vi "check_boc_rms_amplitude_char.vi"(8 "error in (no error)":errorcluster, 9 "Amplitude (1.0 Vpp)":dbl[](array[numeric]) format="%#.4f", 10 "Frequency (Hz)":dbl=1.0 format="%#.4f", 11 "app_data in":T2) -> (0 "error out":errorcluster, 1 "meas":dbl[][](array[numeric]), 2 "boc_data":sgl[][](array[numeric]), 3 "app_data_out":T2)   [LabVIEW 2017]
uses:
  controls/app_data.ctl
  controls/instruments.ctl
  Unicorn Labview Library/Control/unicorn_Param.ctl
  Unicorn Labview Library/Control/unicorn_conn.ctl
  Unicorn Labview Library/Control/unicorn_JSON.ctl
  Unicorn Labview Library/Control/unicorn_ParamInt.ctl
  Unicorn Labview Library/Control/unicorn_Telemetry.ctl
  Unicorn Labview Library/Control/unicorn_Table.ctl
  Unicorn Labview Library/Control/unicorn_ParamFloat.ctl
  controls/attenuator_dB.ctl
  Unicorn Labview Library/Unicorn Library.lvlib
panel:
  out "Attenuator(dB)":T1
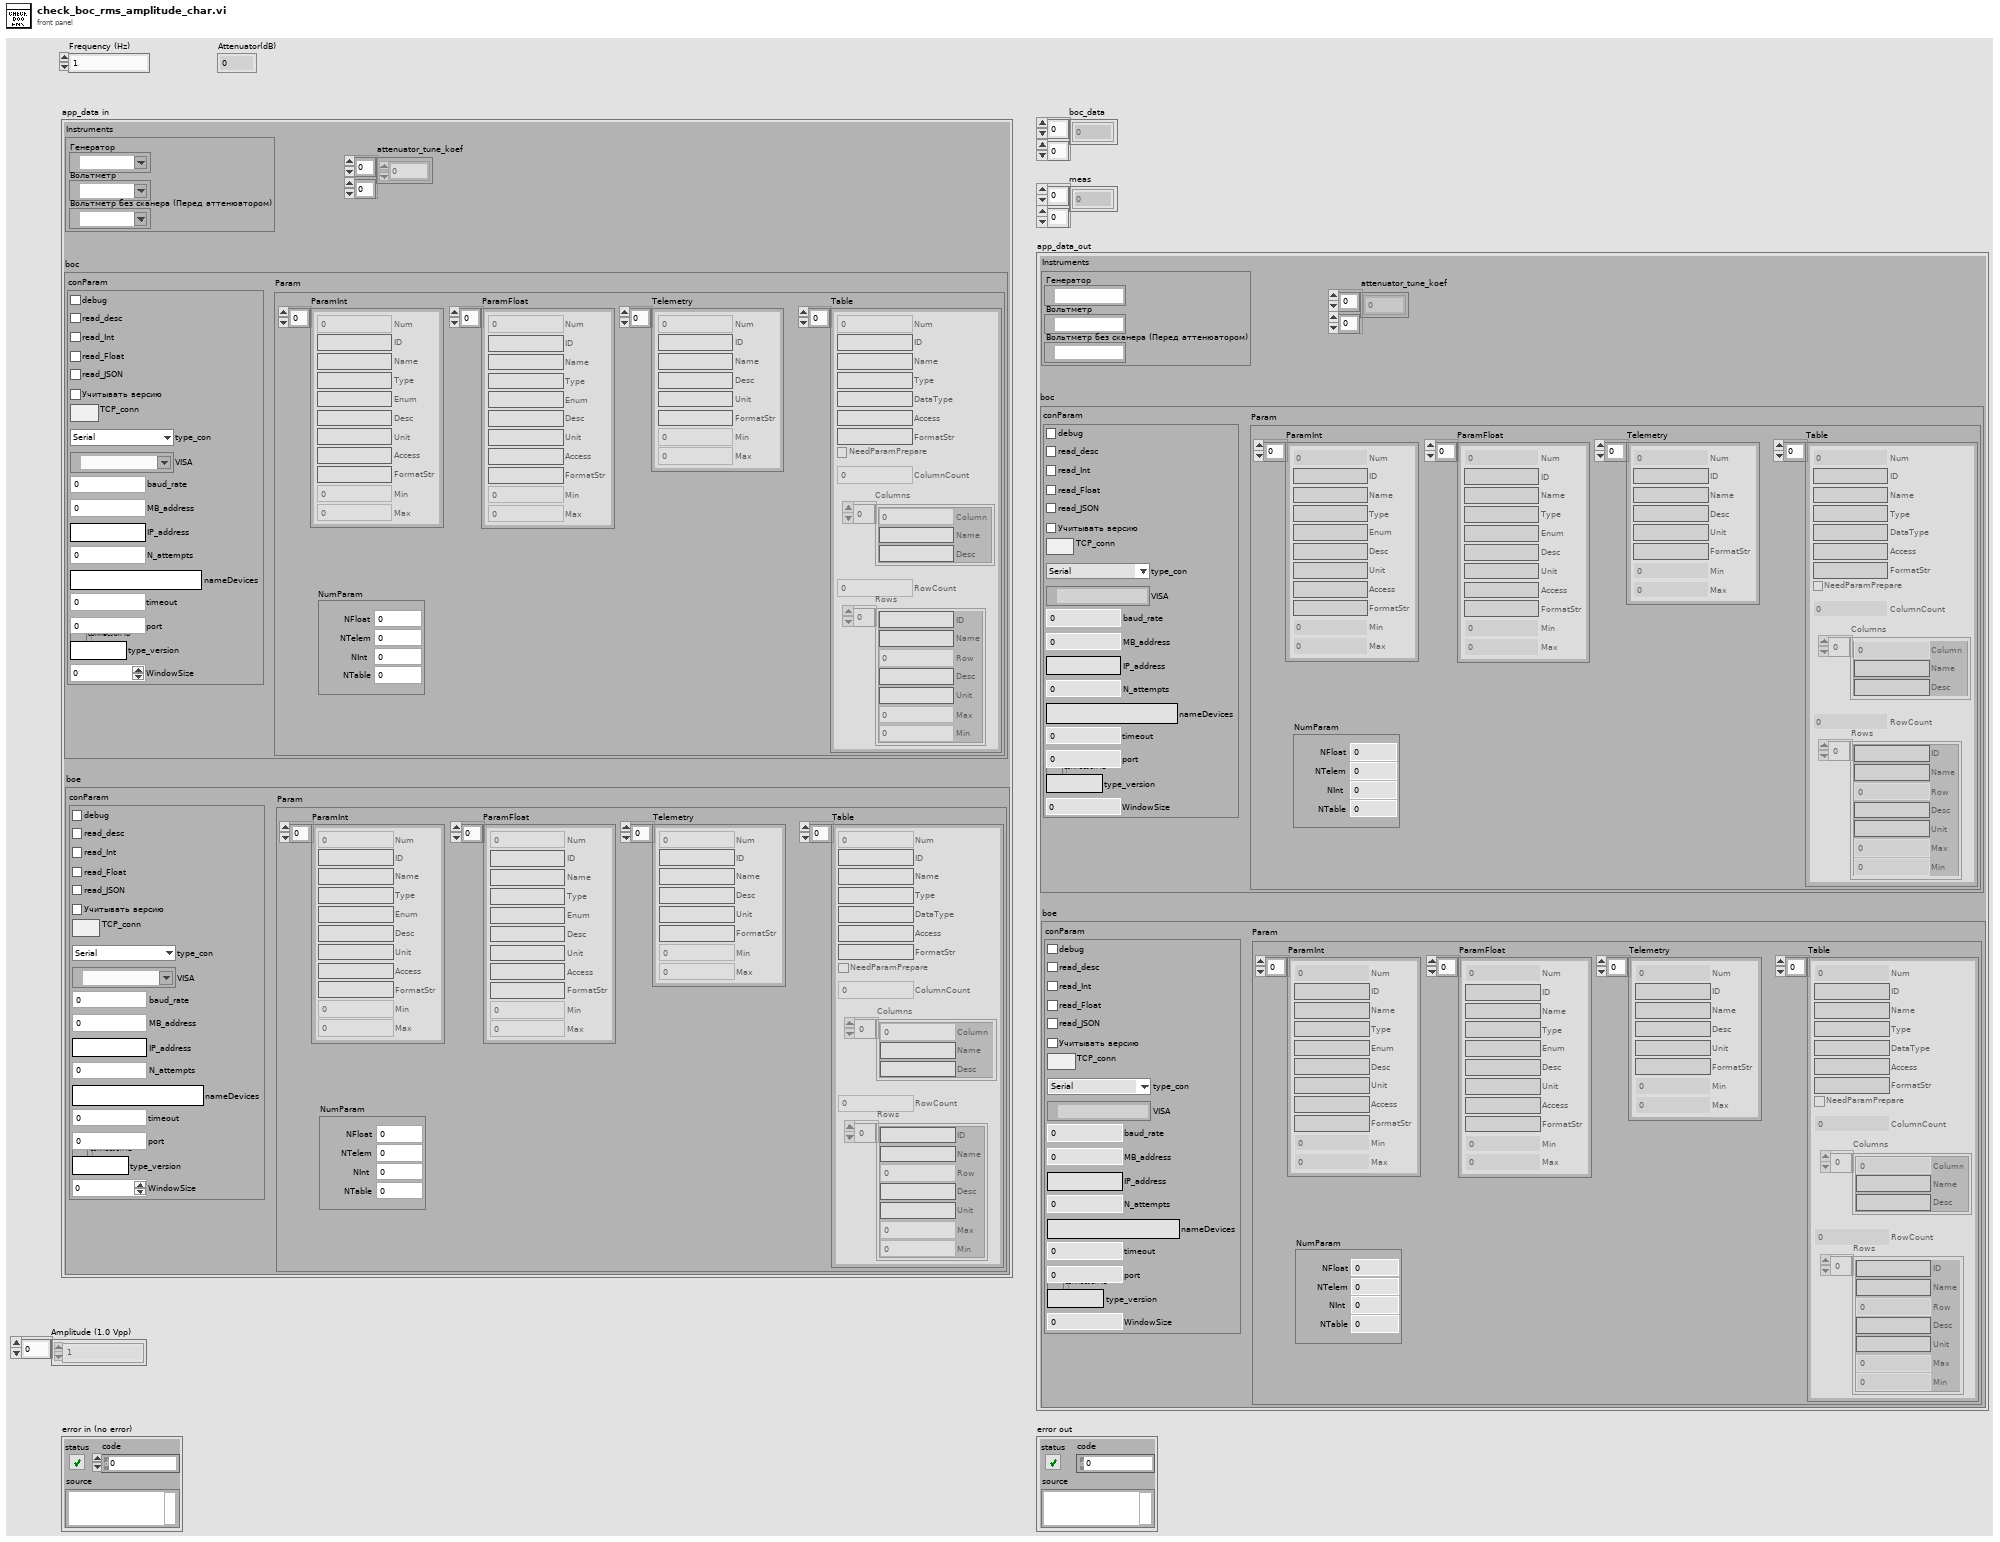
[diagram p1: front panel]
types:
  T1 = typedef "attenuator_dB.ctl" = enum16{"0", "20", "40", "60"}
  T2 = typedef "app_data.ctl" = cluster{"Instruments":T3, "boc":T4, "boe":T4, "attenuator_tune_koef":dbl[][]}
  T3 = typedef "instruments.ctl" = cluster{"generator":refnum<visa-resource-name>, "voltment_with_scaner":refnum<visa-resource-name>, "voltment_without_scaner":refnum<visa-resource-name>}
  T4 = typedef "Unicorn Library.lvlib/unicorn_Param.ctl" = cluster{"conParam":T5, "Param":T6}
  T5 = typedef "Unicorn Library.lvlib/unicorn_conn.ctl" = cluster{"ReadIntParam":bool, "ReadDescrParam":bool, "ReadFloatParam":bool, "debug":bool, "ReadJSON":bool, "IP_address":string, "N_attempts":i32, "type_con":enum16{"Serial", "TCP"}, "MB_address":i32, "VISA":refnum<visa-resource-name>, "connection ID":refnum<k5>, "nameDevices":string, "timeout":i32, "port":u16, "type_version":string, "baud_rate":u32, "VersionControl":bool, "TCP_conn":bool, "WindowSize":i32}
  T6 = typedef "Unicorn Library.lvlib/unicorn_JSON.ctl" = cluster{"NumParam":cluster{"NTelem":i32, "NInt":i32, "NFloat":i32, "NTable":i32}, "ParamInt":T7, "Telemetry":T8, "Table":T9, "ParamFloat":T10}
  T7 = typedef "Unicorn Library.lvlib/unicorn_ParamInt.ctl" = cluster{"ID":string, "Num":i32, "Name":string, "Type":string, "Enum":string, "Desc":string, "Unit":string, "Access":string, "FormatStr":string, "Min":i32, "Max":i32}[]
  T8 = typedef "Unicorn Library.lvlib/unicorn_Telemetry.ctl" = cluster{"ID":string, "Num":i32, "Name":string, "Desc":string, "Unit":string, "FormatStr":string, "Min":i32, "Max":i32}[]
  T9 = typedef "Unicorn Library.lvlib/unicorn_Table.ctl" = cluster{"Num":i32, "Access":string, "ColumnCount":i32, "NeedParamPrepare":bool, "Columns":cluster{"Column":i32, "Desc":string, "Name":string}[], "DataType":string, "FormatStr":string, "ID":string, "Name":string, "RowCount":i32, "Rows":cluster{"Desc":string, "ID":string, "Max":i32, "Min":i32, "Name":string, "Row":i32, "Unit":string}[], "Type":string}[]
  T10 = typedef "Unicorn Library.lvlib/unicorn_ParamFloat.ctl" = cluster{"ID":string, "Num":i32, "Name":string, "Type":string, "Enum":string, "Desc":string, "Unit":string, "Access":string, "FormatStr":string, "Min":i32, "Max":i32}[]
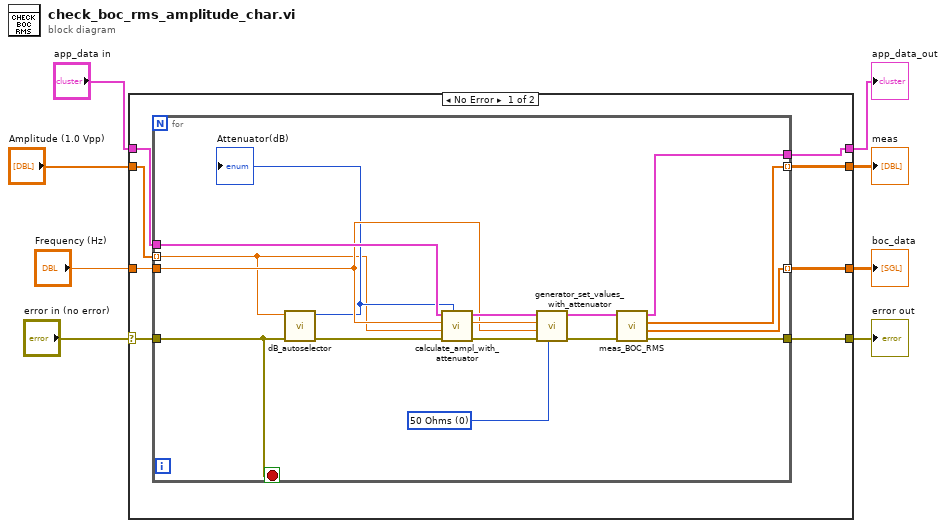
[diagram p0: block diagram]
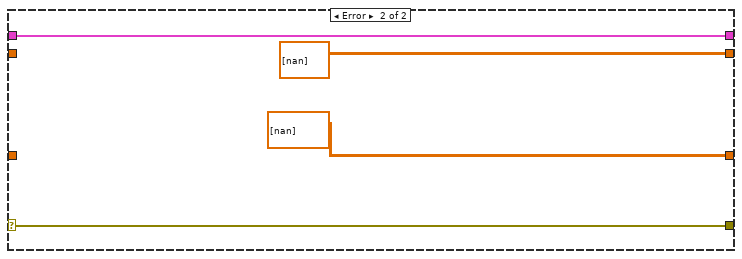
[diagram p2: hidden frame]
diagram:
  n1 = case shown="No Error" "error in (no error)" {
    selector: "error in (no error)" -> [w9 w36]
    tunnel: [w16 dbl[][] [[nan]] ("meas")] -> w8
    tunnel: [w15 sgl[][] [[nan]] ("boc_data")] -> w7
    tunnel: [w14 w36] -> w6
    tunnel: [w13 w35] -> w5
    tunnel: "Amplitude (1.0 Vpp)" -> [w12 _]
    tunnel: "app_data in" -> [w11 w35]
    tunnel: "Frequency (Hz)" -> [w10 _]
    frame No Error {
      n2 = for {
        tunnel: [w28] -> w16 mode=indexing
        tunnel: [w27] -> w15 mode=indexing
        tunnel: w9 -> [w17]
        tunnel: [w29] -> w14
        tunnel: w11 -> [w26]
        tunnel: [w30] -> w13
        tunnel: w12 -> [w19] mode=indexing
        tunnel: w10 -> [w21]
        stop <- w17 stop-if-true
        w22 = u16 0 items=["50 Ohms", "High Impedance"] ("Impedance (0: 50 Ohms)")
        n3 = call "dB_autoselector.vi"("error_in"=w17, "Amplitude"=w19) -> ("error_out"=w18:errorcluster, "Attenuator(dB)"=w20:T1)  [unwired: 8 in]
        "Attenuator(dB)" <- w20
        n4 = call "calculate_ampl_with_attenuator.vi"("Attenuator(dB)"=w20, "error in"=w18, "Amplitude_in"=w19, "frequency"=w21, "app_data in in"=w26) -> ("error out"=w25:errorcluster, "Amplitude_out"=w24:dbl, "app_data out"=w23:T2)  [unwired: 4 in]
        n5 = call "generator_set_values_with_attenuator.vi"("Impedance (0: 50 Ohms)"=w22, "error in (no error)"=w25, "Frequency (1000 Hz)"=w21, "Amplitude (1.0 Vpp)"=w24, "app_data"=w23) -> ("error out"=w31:errorcluster, "output cluster"=w32:T2)  [unwired: 5 in]
        n6 = call "meas_BOC_RMS.vi"("error in (no error)"=w31, "output cluster in"=w32) -> ("error out"=w29:errorcluster, "boc_data"=w27:sgl[], "meas"=w28:dbl[], "output cluster out"=w30:T2)  [unwired: 6 in]
      }
    }
    frame Error {
    }
  }
  "meas" <- w8
  "boc_data" <- w7
  "error out" <- w6
  "app_data_out" <- w5
